vi "Turn OFF SwitchHtr.vi"(8 "error in (no error)":errorcluster, 11 "Turn ON / OFF":bool) -> (0 "error out":errorcluster, 2 "Z-coil HTR status":bool, 3 "Y-coil HTR status":bool)   [LabVIEW 2013]
uses:
  config.vi
panel:
  # "! ZERO field first by running \n\"magnet ramp to field vector.vi\" !"
  # "If switch heaters are found ON (OFF), they are switched OFF (ON) and we wait 20sec.\nIf LHe-level drops below 56%, external \nrampdown mode will be entered,\neven if H=0. HTRs will turn ON & LHe consumption will rise. Also, executing this .vi will yield error. \nTherefore: \na) switch off power supplies\nb) switch off 430 controllers"
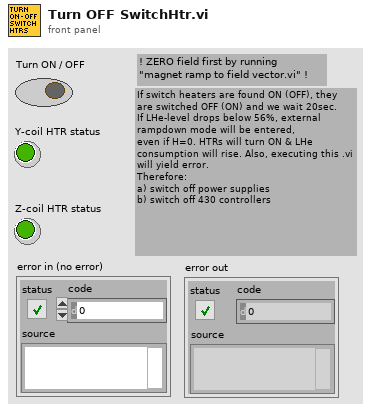
[diagram p1: front panel]
types:
  T1 = cluster{"GPIB address":i16, "GPIB bus":i16, "connection ID":refnum<k5>, "IP":string, "Active Comm Interface":u16, "Serial Port":refnum<visa-resource-name>, "Programmer Type":u16}
  T2 = cluster{"error":bool, "code":i32, "source":string}
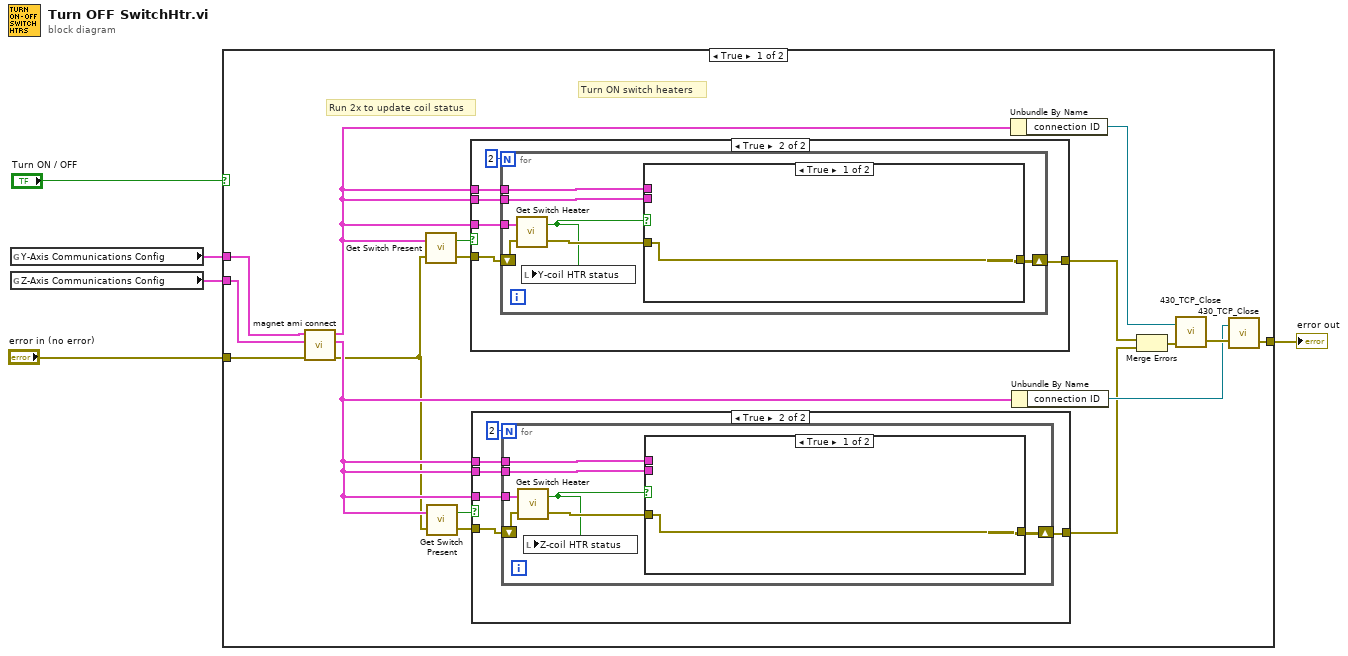
[diagram p0: block diagram]
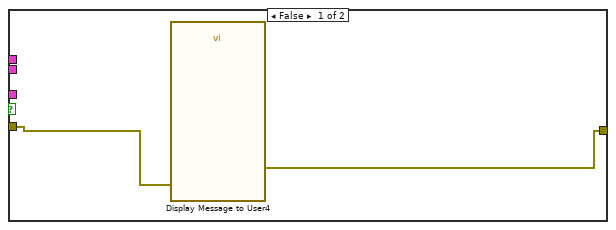
[diagram p2: hidden frame]
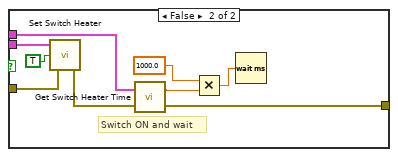
[diagram p3: hidden frame]
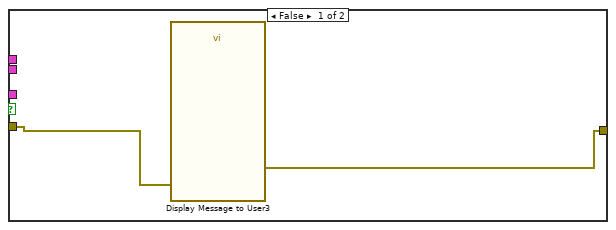
[diagram p4: hidden frame]
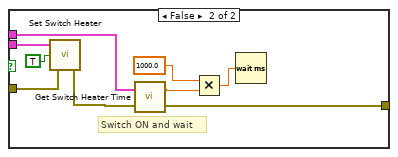
[diagram p5: hidden frame]
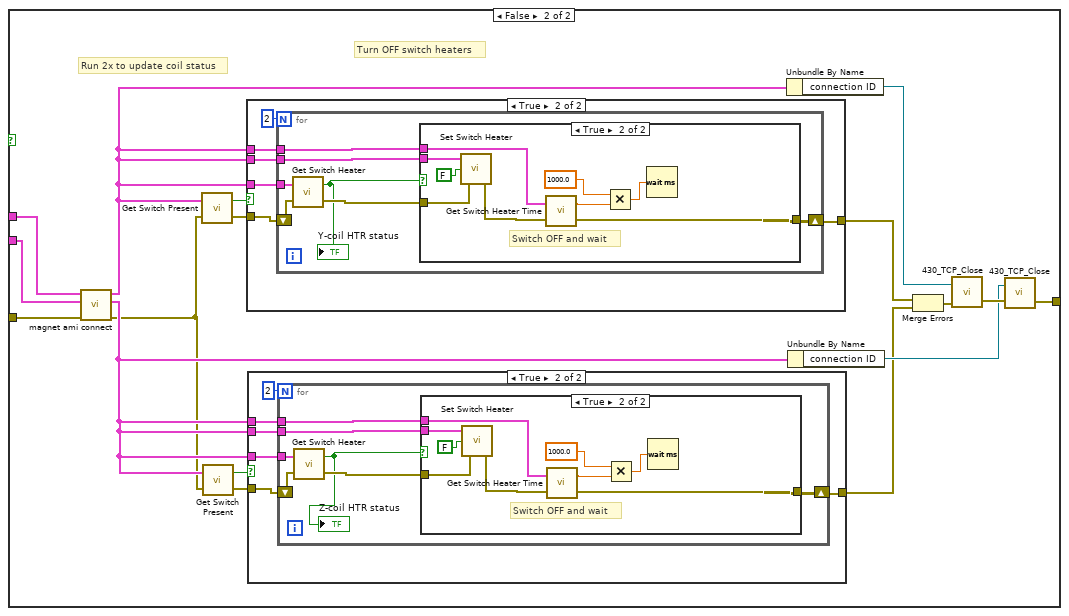
[diagram p6: hidden frame]
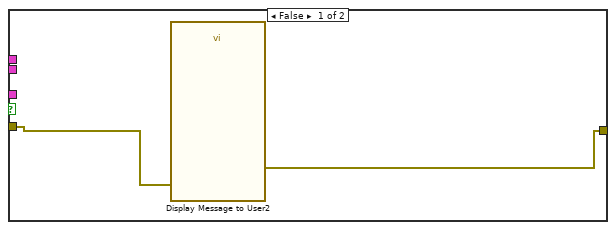
[diagram p7: hidden frame]
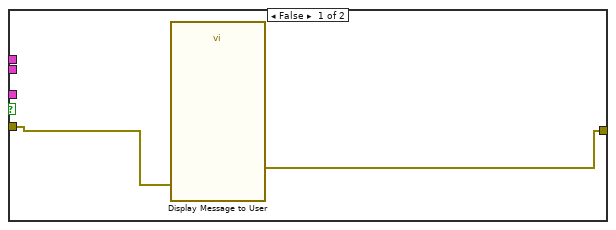
[diagram p9: hidden frame]
diagram:
  n1 = global read "config.vi" "Y-Axis Communications Config"() -> (w2:T1)
  n2 = global read "config.vi" "Z-Axis Communications Config"() -> (w1:T1)
  n3 = case shown="True" "Turn ON / OFF" {
    tunnel: "error in (no error)" -> [w8 w87]
    tunnel: [w9 w81] -> w4
    tunnel: w2 -> [w6 w74]
    tunnel: w1 -> [w7 w73]
    frame True {
      # "Turn ON switch heaters"
      # "Run 2x to update coil status"
      n4 = call "magnet ami connect.vi"("error in (no error)"=w8, "Z-Axis Communications Config"=w7, "Y-Axis Communications Config"=w6) -> ("error out"=w12:errorcluster, "Z-Axis Communications Config Out"=w13:T1, "Y-Axis Communications Config Out"=w18:T1)  [unwired: 6 in]
      n5 = call <userlib>:"Get Switch Present.vi"("error in"=w12, "Communications Config"=w18) -> ("error out"=w19:T2, "Switch Present?"=w20:bool)
      n6 = call <userlib>:"Get Switch Present.vi"("error in"=w12, "Communications Config"=w13) -> ("error out"=w16:T2, "Switch Present?"=w17:bool)
      n7 = case shown="True" w20 {
        tunnel: w18 -> [_ w55]
        tunnel: w18 -> [_ w54]
        tunnel: w18 -> [_ w53]
        tunnel: w19 -> [w49 w52]
        tunnel: [w48 w50] -> w11
        frame False {
          n8 = call "Display Message to User3"("error in (no error)"=w49) -> ("error out"=w48:errorcluster)  [unwired: 9 in, 1 out]
        }
        frame True {
          n9 = for {
            N: 2 -> [_]
            tunnel: w55 -> [w62]
            tunnel: w54 -> [w61]
            tunnel: w53 -> [w60]
            shift-right: [w57] -> w50
            shift-left: w52 -> [w59]
            n10 = call <userlib>:"Get Switch Heater.vi"("error in"=w59, "Communications Config"=w62) -> ("error out"=w58:T2, "Switch Heater Indicator"=w56:bool)
            n11 = local write "Y-coil HTR status"(w56) -> ()
            n12 = case shown="True" w56 {
              tunnel: w61 -> [_ w71]
              tunnel: w60 -> [_ w70]
              tunnel: w58 -> [w63 w69]
              tunnel: [w63 w68] -> w57
              frame True {
              }
              frame False {
                # "Switch ON and wait"
                n13 = call <userlib>:"Set Switch Heater.vi"("error in"=w69, "Switch Heater Control"=TRUE, "Communications Config"=w71) -> ("error out"=w72:T2)
                n14 = call <userlib>:"Get Switch Heater Time.vi"("error in"=w72, "Communications Config"=w70) -> ("error out"=w68:T2, "Switch Heating Time (secs)"=w66:dbl)
                n15 = Multiply(x=1000.0 ("y"), y=w66) -> (x*y=w64:dbl)
                n16 = Wait (ms)(milliseconds to wait=w64) -> ()  [unwired: 1 out]
              }
            }
          }
        }
      }
      n17 = case shown="True" w17 {
        tunnel: w13 -> [_ w30]
        tunnel: w13 -> [_ w29]
        tunnel: w13 -> [_ w28]
        tunnel: w16 -> [w24 w27]
        tunnel: [w23 w25] -> w10
        frame False {
          n18 = call "Display Message to User4"("error in (no error)"=w24) -> ("error out"=w23:errorcluster)  [unwired: 9 in, 1 out]
        }
        frame True {
          n19 = for {
            N: 2 -> [_]
            tunnel: w30 -> [w37]
            tunnel: w29 -> [w36]
            tunnel: w28 -> [w35]
            shift-right: [w32] -> w25
            shift-left: w27 -> [w34]
            n20 = call <userlib>:"Get Switch Heater.vi"("error in"=w34, "Communications Config"=w37) -> ("error out"=w33:T2, "Switch Heater Indicator"=w31:bool)
            n21 = local write "Z-coil HTR status"(w31) -> ()
            n22 = case shown="True" w31 {
              tunnel: w36 -> [_ w46]
              tunnel: w35 -> [_ w45]
              tunnel: w33 -> [w38 w44]
              tunnel: [w38 w43] -> w32
              frame True {
              }
              frame False {
                # "Switch ON and wait"
                n23 = call <userlib>:"Set Switch Heater.vi"("error in"=w44, "Switch Heater Control"=TRUE, "Communications Config"=w46) -> ("error out"=w47:T2)
                n24 = call <userlib>:"Get Switch Heater Time.vi"("error in"=w47, "Communications Config"=w45) -> ("error out"=w43:T2, "Switch Heating Time (secs)"=w41:dbl)
                n25 = Multiply(x=1000.0 ("y"), y=w41) -> (x*y=w39:dbl)
                n26 = Wait (ms)(milliseconds to wait=w39) -> ()  [unwired: 1 out]
              }
            }
          }
        }
      }
      n27 = Unbundle By Name(w18) -> ("connection ID"=w22:refnum<k5>)
      n28 = Unbundle By Name(w13) -> ("connection ID"=w14:refnum<k5>)
      n29 = Merge Errors(w11, w10) -> (w21:errorcluster)
      n30 = call <userlib>:"430_TCP_Close.vi"("error in (no error)"=w21, "connection ID"=w22) -> ("error out"=w15:errorcluster)  [unwired: 1 out]
      n31 = call <userlib>:"430_TCP_Close.vi"("error in (no error)"=w15, "connection ID"=w14) -> ("error out"=w9:errorcluster)  [unwired: 1 out]
    }
    frame False {
      # "Turn OFF switch heaters"
      # "Run 2x to update coil status"
      n32 = call "magnet ami connect.vi"("error in (no error)"=w87, "Z-Axis Communications Config"=w73, "Y-Axis Communications Config"=w74) -> ("error out"=w77:errorcluster, "Z-Axis Communications Config Out"=w78:T1, "Y-Axis Communications Config Out"=w84:T1)  [unwired: 6 in]
      n33 = call <userlib>:"Get Switch Present.vi"("error in"=w77, "Communications Config"=w84) -> ("error out"=w85:T2, "Switch Present?"=w86:bool)
      n34 = call <userlib>:"Get Switch Present.vi"("error in"=w77, "Communications Config"=w78) -> ("error out"=w82:T2, "Switch Present?"=w83:bool)
      n35 = case shown="True" w86 {
        tunnel: w84 -> [_ w122]
        tunnel: w84 -> [_ w121]
        tunnel: w84 -> [_ w120]
        tunnel: w85 -> [w116 w119]
        tunnel: [w115 w117] -> w76
        frame False {
          n36 = call "Display Message to User"("error in (no error)"=w116) -> ("error out"=w115:errorcluster)  [unwired: 9 in, 1 out]
        }
        frame True {
          n37 = for {
            N: 2 -> [_]
            tunnel: w122 -> [w129]
            tunnel: w121 -> [w128]
            tunnel: w120 -> [w127]
            shift-right: [w124] -> w117
            shift-left: w119 -> [w126]
            n38 = call <userlib>:"Get Switch Heater.vi"("error in"=w126, "Communications Config"=w129) -> ("error out"=w125:T2, "Switch Heater Indicator"=w123:bool)
            "Y-coil HTR status" <- w123
            n39 = case shown="True" w123 {
              tunnel: w128 -> [_ w138]
              tunnel: w127 -> [_ w137]
              tunnel: w125 -> [w130 w136]
              tunnel: [w130 w135] -> w124
              frame False {
              }
              frame True {
                # "Switch OFF and wait"
                n40 = call <userlib>:"Set Switch Heater.vi"("error in"=w136, "Switch Heater Control"=FALSE, "Communications Config"=w138) -> ("error out"=w139:T2)
                n41 = call <userlib>:"Get Switch Heater Time.vi"("error in"=w139, "Communications Config"=w137) -> ("error out"=w135:T2, "Switch Heating Time (secs)"=w133:dbl)
                n42 = Multiply(x=1000.0 ("y"), y=w133) -> (x*y=w131:dbl)
                n43 = Wait (ms)(milliseconds to wait=w131) -> ()  [unwired: 1 out]
              }
            }
          }
        }
      }
      n44 = case shown="True" w83 {
        tunnel: w78 -> [_ w97]
        tunnel: w78 -> [_ w96]
        tunnel: w78 -> [_ w95]
        tunnel: w82 -> [w91 w94]
        tunnel: [w90 w92] -> w75
        frame False {
          n45 = call "Display Message to User2"("error in (no error)"=w91) -> ("error out"=w90:errorcluster)  [unwired: 9 in, 1 out]
        }
        frame True {
          n46 = for {
            N: 2 -> [_]
            tunnel: w97 -> [w104]
            tunnel: w96 -> [w103]
            tunnel: w95 -> [w102]
            shift-right: [w99] -> w92
            shift-left: w94 -> [w101]
            n47 = call <userlib>:"Get Switch Heater.vi"("error in"=w101, "Communications Config"=w104) -> ("error out"=w100:T2, "Switch Heater Indicator"=w98:bool)
            "Z-coil HTR status" <- w98
            n48 = case shown="True" w98 {
              tunnel: w103 -> [_ w113]
              tunnel: w102 -> [_ w112]
              tunnel: w100 -> [w105 w111]
              tunnel: [w105 w110] -> w99
              frame False {
              }
              frame True {
                # "Switch OFF and wait"
                n49 = call <userlib>:"Set Switch Heater.vi"("error in"=w111, "Switch Heater Control"=FALSE, "Communications Config"=w113) -> ("error out"=w114:T2)
                n50 = call <userlib>:"Get Switch Heater Time.vi"("error in"=w114, "Communications Config"=w112) -> ("error out"=w110:T2, "Switch Heating Time (secs)"=w108:dbl)
                n51 = Multiply(x=1000.0 ("y"), y=w108) -> (x*y=w106:dbl)
                n52 = Wait (ms)(milliseconds to wait=w106) -> ()  [unwired: 1 out]
              }
            }
          }
        }
      }
      n53 = Unbundle By Name(w84) -> ("connection ID"=w89:refnum<k5>)
      n54 = Unbundle By Name(w78) -> ("connection ID"=w79:refnum<k5>)
      n55 = Merge Errors(w76, w75) -> (w88:errorcluster)
      n56 = call <userlib>:"430_TCP_Close.vi"("error in (no error)"=w88, "connection ID"=w89) -> ("error out"=w80:errorcluster)  [unwired: 1 out]
      n57 = call <userlib>:"430_TCP_Close.vi"("error in (no error)"=w80, "connection ID"=w79) -> ("error out"=w81:errorcluster)  [unwired: 1 out]
    }
  }
  "error out" <- w4
